vi "_value_view.vi"(8 "error in (no error)":errorcluster, 11 "Value in":refnum<class "Value.lvclass">) -> (0 "error out":errorcluster, 2 "Val View":T1={"Value"=0.0, "grad"=0.0, "label"="", "operation"=enum."add", "serial"=0}, 3 "Value out":refnum<class "Value.lvclass">)   [LabVIEW 2023, in "LabGRAD.lvlib" / "Value.lvclass"]
uses:
  Value.lvclass
  value view.ctl
  UiObjects/numeric value control.ctl
  UiObjects/string control.ctl
  operation.ctl
  Value.lvclass/Value.ctl
  UiObjects/UiObjects.lvclass
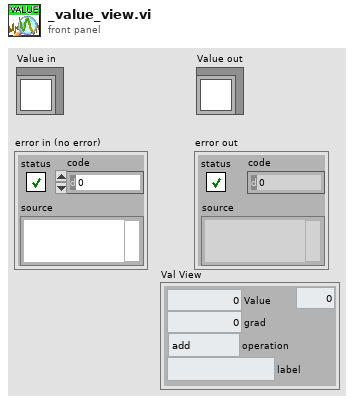
[diagram p1: front panel]
types:
  T1 = typedef "LabGRAD.lvlib/Value.lvclass/value view.ctl" = cluster{"Value":T2, "grad":T2, "label":T3, "operation":T4, "serial":u32}
  T2 = typedef "UiObjects.lvlib/UiObjects.lvclass/numeric value control.ctl" = dbl
  T3 = typedef "UiObjects.lvlib/UiObjects.lvclass/string control.ctl" = string
  T4 = typedef "LabGRAD.lvlib/Value.lvclass/operation.ctl" = enum16{"nop", "add", "subtract", "power", "multiply", "divide", "tanh"}
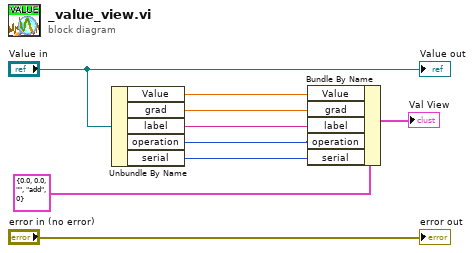
[diagram p0: block diagram]
diagram:
  n1 = Unbundle By Name("Value in") -> ("Value"=w5:T2, "grad"=w4:T2, "label"=w3:T3, "operation"=w2:T4, "serial"=w1:u32)
  n2 = Bundle By Name(cluster=T1 {"Value"=0.0, "grad"=0.0, "label"="", "operation"=enum."add", "serial"=0} ("Cluster"), "Value"=w5, "grad"=w4, "label"=w3, "operation"=w2, "serial"=w1) -> (→"Val View":T1)
  "error out" <- "error in (no error)"
  "Value out" <- "Value in"
